vi "Check on event.vi"(7 "Event threshold (0,02V)":dbl=0.02 min=0.0 max=0.5 step=0.01 format="%#_6gV", 8 "Error In":errorcluster, 9 "YPR data":dbl[](array[numeric])=[0.0, 0.0, 0.0, 0.0, 0.0, 0.0, 0.0, 0.0, 0.0, 0.0, 0.0, 0.0], 10 "Strain data":dbl[](array[numeric])=[0.0, 0.0, 0.0, 0.0, 0.0, 0.0, 0.0, 0.0, 0.0, 0.0, 0.0, 0.0], 11 "Event cluster in":T1) -> (0 "Error Out":errorcluster, 1 "event ongoing":bool, 2 "new event finished":bool, 3 "Event cluster":T1)   [LabVIEW 2016]
uses:
  Typedef/Event cluster.ctl
  Typedef/SVM predict class.ctl
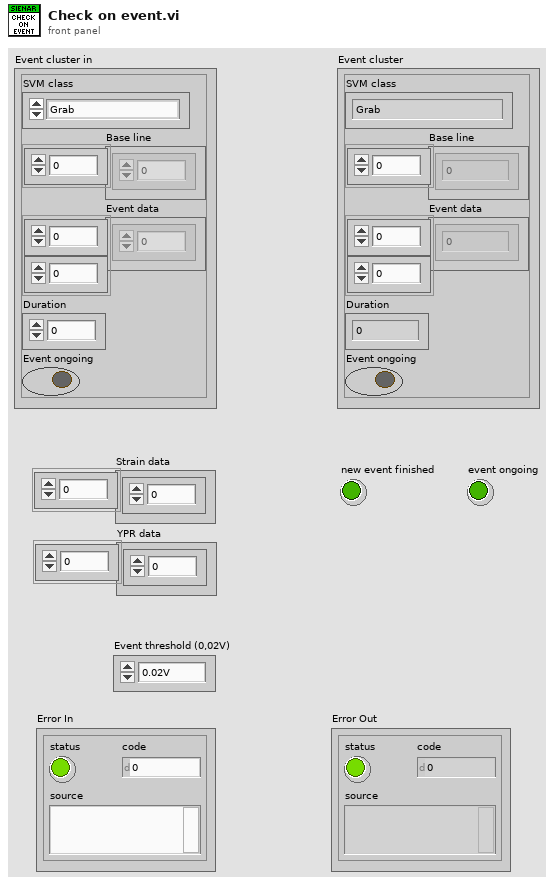
[diagram p1: front panel]
types:
  T1 = typedef "Event cluster.ctl" = cluster{"SVM class":T2, "Base line":dbl[], "Event data":dbl[][], "Duration":dbl, "Event ongoing":bool}
  T2 = typedef "SVM predict class.ctl" = enum16{"Grab", "Grab release", "Hand flexion", "Hand flexion release", "Hand extension", "Hand extension release", "Tap", "Swipe_CW", "Swipe_CCW"}
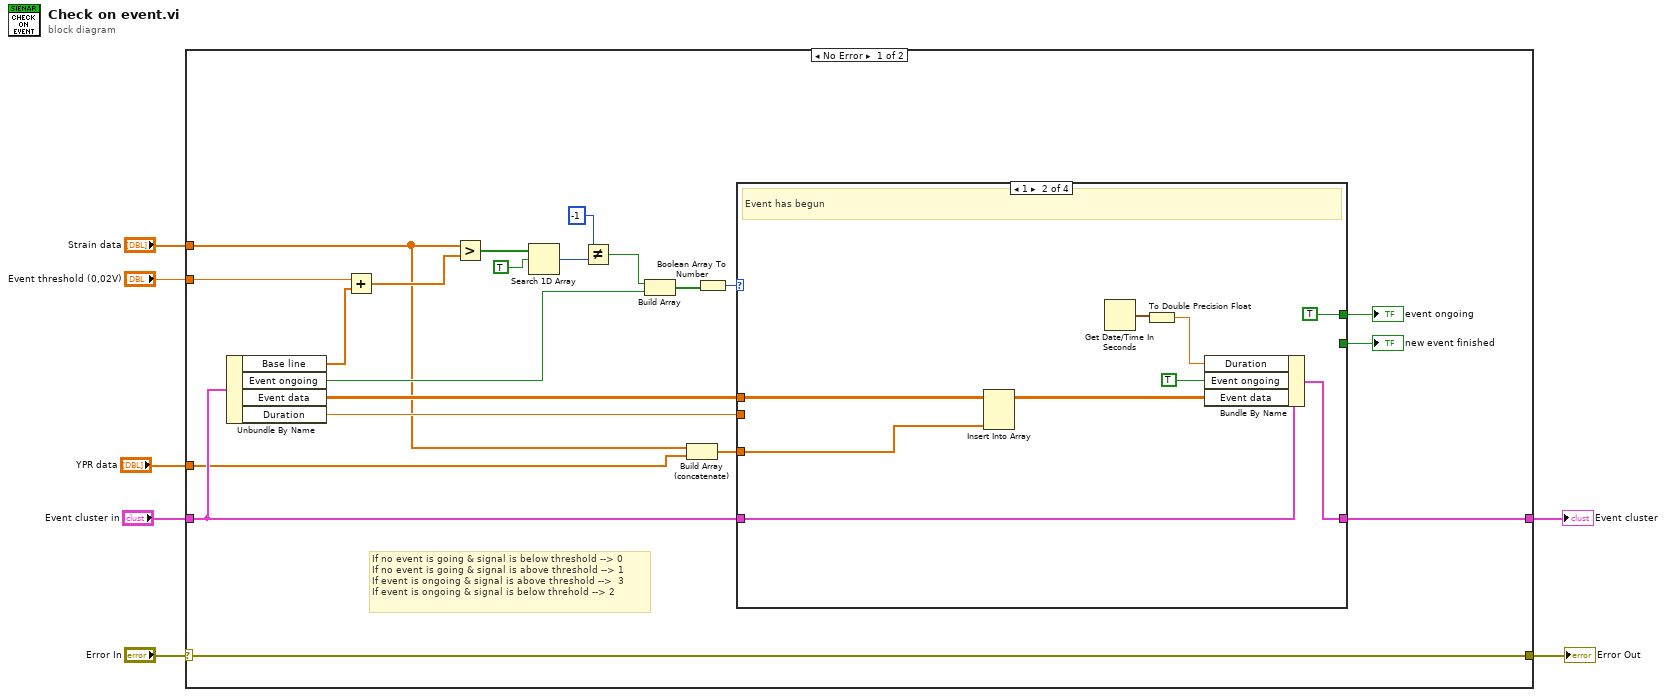
[diagram p0: block diagram]
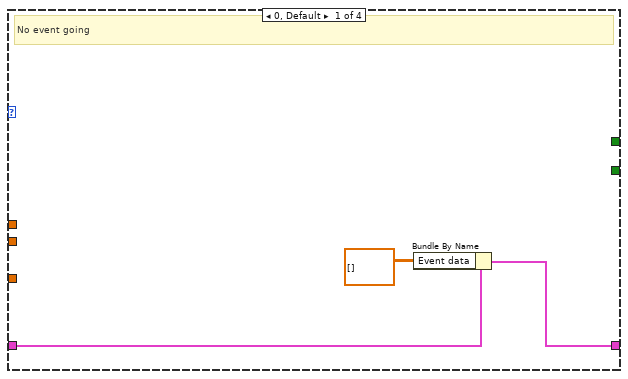
[diagram p2: hidden frame]
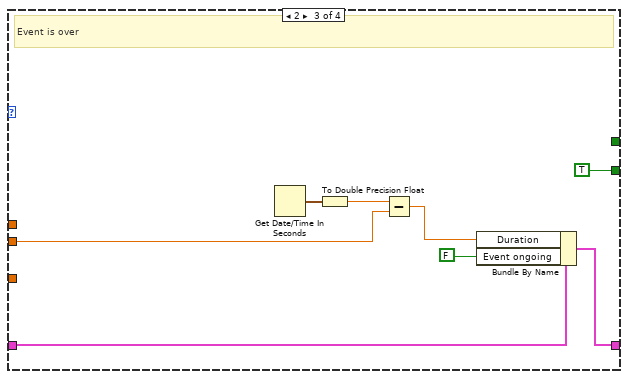
[diagram p3: hidden frame]
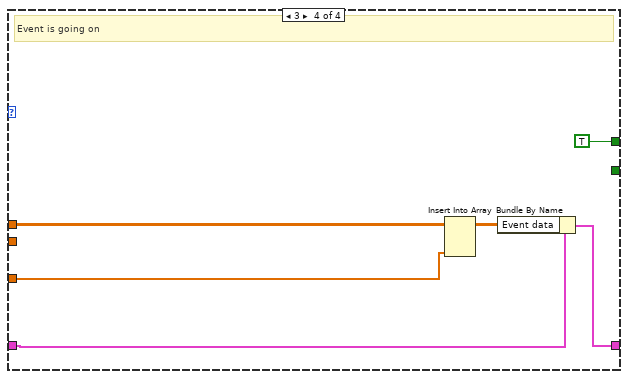
[diagram p4: hidden frame]
diagram:
  n1 = case shown="No Error" "Error In" {
    selector: "Error In" -> [w14 w55]
    tunnel: "Event cluster in" -> [w17 w56]
    tunnel: "Event threshold (0,02V)" -> [w24 _]
    tunnel: "Strain data" -> [w11 _]
    tunnel: [w16 w56] -> w2
    tunnel: [w14 w55] -> w3
    tunnel: "YPR data" -> [w10 _]
    frame No Error {
      # "If no event is going & signal is below threshold --> 0\nIf no event is going & signal is above threshold --> 1\nIf event is ongoing & signal is above threshold -->  3\nIf event is ongoing & signal is below threhold --> 2"
      n2 = Unbundle By Name(w17) -> ("Base line"=w28:dbl[], "Event ongoing"=w21:bool, "Event data"=w15:dbl[][], "Duration"=w13:dbl)
      n3 = Add(x=w24, y=w28) -> (x+y=w27:dbl[])
      n4 = Greater?(x=w11, y=w27) -> (0:w25:bool[])
      n5 = Search 1D Array(1D array=w25, element=TRUE) -> (index of element=w23:i32)  [unwired: 1 in]
      n6 = Not Equal?(x=-1 ("y"), y=w23) -> (x != y?=w20:bool)
      n7 = Build Array(w20, w21) -> (w19:bool[])
      n8 = Build Array (concatenate)(w11, w10) -> (w9:dbl[])
      n9 = Boolean Array To Number(Boolean array=w19) -> (number=w18:u32)
      n10 = case shown="1" w18 {
        tunnel: w17 -> [w31 w40 w47 w52]
        tunnel: [w30 w39 w46 w53] -> w16
        tunnel: w15 -> [_ w37 _ w54]
        tunnel: w13 -> [_ _ w43 _]
        tunnel: [_ _ TRUE _] -> w12
        tunnel: w9 -> [_ w33 _ w50]
        tunnel: [_ TRUE _ TRUE] -> w8
        frame 0, Default {
          # "No event going"
          n11 = Bundle By Name(cluster=w31, "Event data"=dbl[][] []) -> (w30:T1)
        }
        frame 1 {
          # "Event has begun"
          n12 = Insert Into Array(array=w37, new element=w33) -> (w36:dbl[][])  [unwired: 2 in]
          n13 = Get Date/Time In Seconds() -> (seconds since 1Jan1904=w35:timestamp)
          n14 = To Double Precision Float(number=w35) -> (double precision float=w34:dbl)
          n15 = Bundle By Name(cluster=w40, "Duration"=w34, "Event ongoing"=TRUE, "Event data"=w36) -> (w39:T1)
        }
        frame 2 {
          # "Event is over"
          n16 = Get Date/Time In Seconds() -> (seconds since 1Jan1904=w45:timestamp)
          n17 = To Double Precision Float(number=w45) -> (double precision float=w44:dbl)
          n18 = Subtract(x=w44, y=w43) -> (x-y=w42:dbl)
          n19 = Bundle By Name(cluster=w47, "Duration"=w42, "Event ongoing"=FALSE) -> (w46:T1)
        }
        frame 3 {
          # "Event is going on"
          n20 = Insert Into Array(array=w54, new element=w50) -> (w51:dbl[][])  [unwired: 2 in]
          n21 = Bundle By Name(cluster=w52, "Event data"=w51) -> (w53:T1)
        }
      }
      "new event finished" <- w12
      "event ongoing" <- w8
    }
    frame Error {
    }
  }
  "Error Out" <- w3
  "Event cluster" <- w2
